vi "NI VeriStand - Set Parameter Value.vi"   [LabVIEW 2020, in "NI_VS ModelManager ExecutionAPI.lvlib"]
doc: "Sets values of model parameters present on the target. You must manually select the polymorphic instance to use."
uses:
  <vilib>/NI VeriStand/Execution/ModelManager/NI_VS ModelManager ExecutionAPI.lvlib
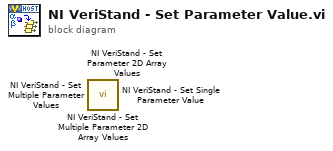
[diagram p0: block diagram]
diagram:
  n1 = call <vilib>:"NI VeriStand - Set Multiple Parameter 2D Array Values.vi"() -> ()  [unwired: 10 in, 2 out]
  n2 = call <vilib>:"NI VeriStand - Set Parameter 2D Array Values.vi"() -> ()  [unwired: 10 in, 2 out]
  n3 = call <vilib>:"NI VeriStand - Set Multiple Parameter Values.vi"() -> ()  [unwired: 10 in, 2 out]
  n4 = call <vilib>:"NI VeriStand - Set Single Parameter Value.vi"() -> ()  [unwired: 10 in, 2 out]
